vi "Error Handling.vi"   [LabVIEW 2019, in "Logger.Error.lvclass"]
uses:
  Logger.Error.lvclass
  <vilib>/Utility/error.llb/Error Cluster From Error Code.vi
  <vilib>/Utility/file.llb/Write Delimited Spreadsheet (string).vi
  <vilib>/ErrorRing/Error Ring.xnode
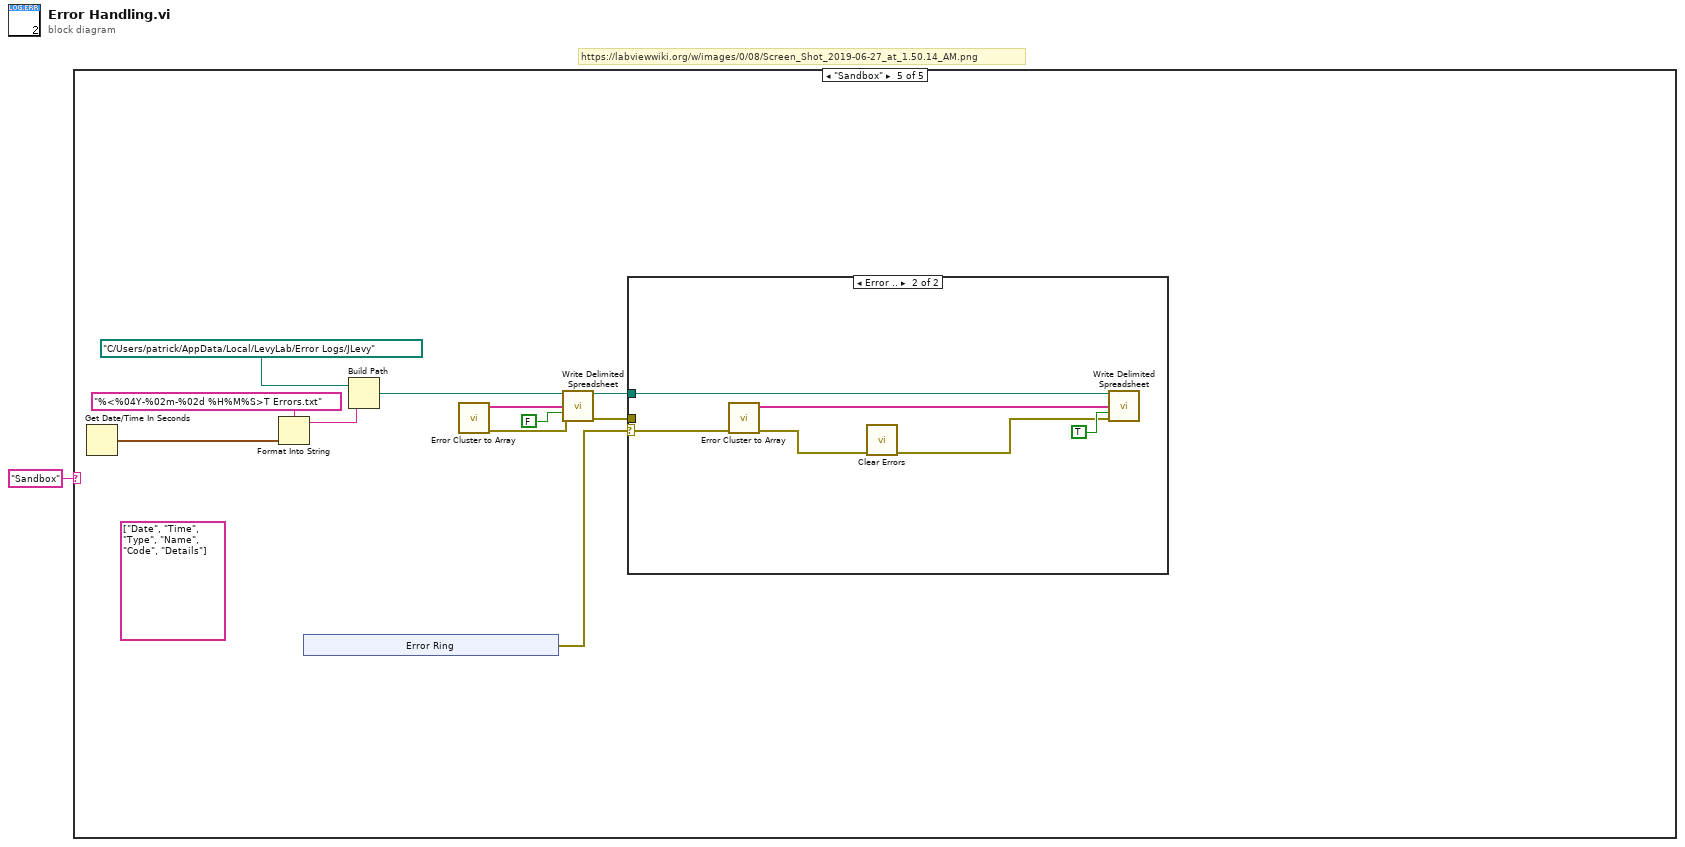
[diagram p0: block diagram]
diagram:
  # "https://labviewwiki.org/w/images/0/08/Screen_Shot_2019-06-27_at_1.50.14_AM.png"
  n1 = case shown="\"Sandbox\"" "Sandbox" {
    frame "Typical", Default {
    }
    frame "Ignore" {
    }
    frame "Retry or Fail" {
    }
    frame "Modifications" {
    }
    frame "Sandbox" {
      (unwired) string[] ["Date", "Time", "Type", "Name", "Code", "Details"] ("string array")
      n2 = Get Date/Time In Seconds() -> (seconds since 1Jan1904=w10:timestamp)
      n3 = Format Into String(format string="%<%04Y-%02m-%02d %H%M%S>T Errors.txt", w10) -> (resulting string=w9:string)  [unwired: 2 in, 1 out]
      n4 = xnode "Error Ring"() -> ("error out"=w12:errorcluster)
      n5 = Build Path(base path=path "C:/Users/patrick/AppData/Local/LevyLab/Error Logs/JLevy" ("file path (dialog if empty)"), name or relative path=w9) -> (appended path=w7:path)
      n6 = call "Error Cluster to Array.vi"() -> ("error out"=w2:errorcluster, "Error Array"=w3:string[])  [unwired: 10 in]
      n7 = call-poly <vilib>:"Write Delimited Spreadsheet.vi"("file path (dialog if empty)"=w7, "1D data"=w3, "append to file? (new file:F)"=FALSE, "error in (no error)"=w2) -> ("new file path (Not A Path if cancelled)"=w5:path, "error out"=w6:errorcluster)  [unwired: 10 in]
      n8 = case shown="Error .." w12 {
        selector: w12 -> [_ w18]
        tunnel: w6 -> [_ _]
        tunnel: w5 -> [_ w16]
        frame No Error {
        }
        frame Error {
          n9 = call "Error Cluster to Array.vi"("error in (no error)"=w18) -> ("error out"=w14:errorcluster, "Error Array"=w17:string[])  [unwired: 9 in]
          n10 = call <vilib>:"Clear Errors.vi"("error in (no error)"=w14) -> ("error out"=w13:errorcluster)  [unwired: 5 in, 1 out]
          n11 = call-poly <vilib>:"Write Delimited Spreadsheet.vi"("file path (dialog if empty)"=w16, "1D data"=w17, "append to file? (new file:F)"=TRUE, "error in (no error)"=w13) -> ()  [unwired: 10 in, 2 out]
        }
      }
    }
  }
